vi "detNbrStepsInProfile.vi"(8 "error in (no error)":errorcluster, 11 "TestMonitor in":refnum<class "TestMonitor.lvclass">) -> (0 "error out":errorcluster, 3 "TestMonitor out":refnum<class "TestMonitor.lvclass">)   [LabVIEW 2015]
uses:
  TestMonitor.lvclass
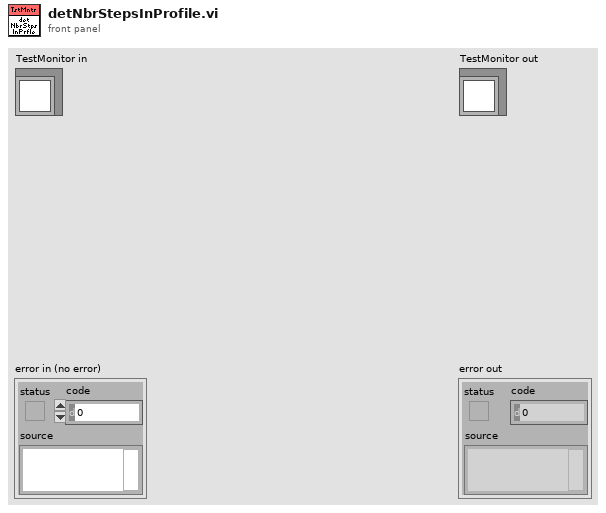
[diagram p1: front panel]
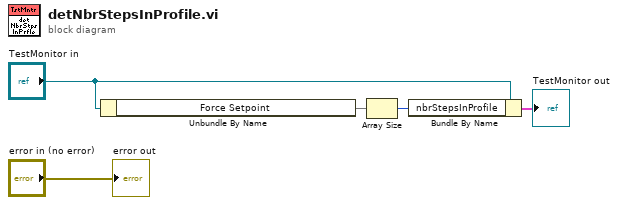
[diagram p0: block diagram]
diagram:
  n1 = Unbundle By Name("TestMonitor in") -> ("Force Setpoint"=w4)
  n2 = Array Size(array=w4) -> (size(s)=w3:i32)
  n3 = Bundle By Name(cluster="TestMonitor in", "nbrStepsInProfile"=w3) -> (→"TestMonitor out":cluster{})
  "error out" <- "error in (no error)"
